vi "fgt get pressure channels Info.vi"(8 "error in (no error)":errorcluster) -> (0 "error out":errorcluster, 3 "Pressure channels info":T1[](array[typedef]) {"indexID" format="%.0x"; "index" format="%.0x"; "position" format="%.0x"; "DeviceSN" format="%.0x"; "firmware" format="%.0x"; "ControllerSN" format="%.0x"})   [LabVIEW 2020, in "fgt_SDK.lvlib"]
doc: "Get total number of initialized pressure channels. It is the sum of all MFCS, MFCS-EZ and FlowEZ pressure controllers"
uses:
  fgt_SDK.lvlib
  TypeDefs/fgt_CHANNEL_INFO.ctl
  TypeDefs/fgt_INSTRUMENT_TYPE.ctl
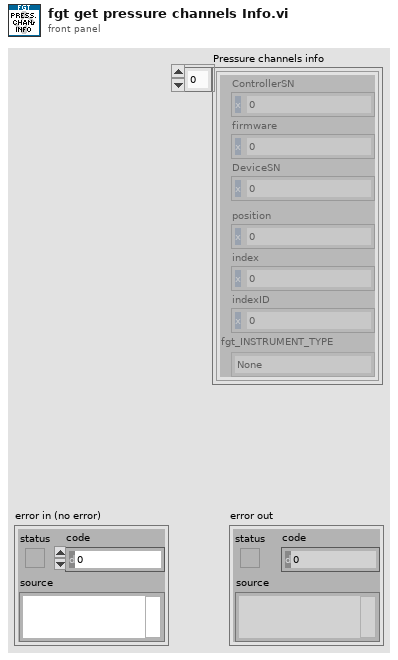
[diagram p1: front panel]
types:
  T1 = typedef "fgt_SDK.lvlib/fgt_CHANNEL_INFO.ctl" = cluster{"ControllerSN":u16, "firmware":u16, "DeviceSN":u16, "position":u32, "index":u32, "indexID":u32, "fgt_INSTRUMENT_TYPE":T2}
  T2 = typedef "fgt_SDK.lvlib/fgt_INSTRUMENT_TYPE.ctl" = enum32{"None", "MFCS", "MFCS_EZ", "FRP", "LineUP", "IPS"}
  T3 = cluster{"ControllerSN":u16, "firmware":u16, "DeviceSN":u16, "Padding":u16, "position":u32, "index":u32, "indexID":u32, "fgt_INSTRUMENT_TYPE":T2}
  T4 = cluster{"ControllerSN":u16, "firmware":u16, "DeviceSN":u16, "Padding":u16, "position":u32, "index":u32, "indexID":u32, "fgt_INSTRUMENT_TYPE":T2}[]
  T5 = typedef "fgt_SDK.lvlib/fgt_STATUS_INFO.ctl" = cluster{"InstrType":T2, "instrSN":u16, "errorCode":u8, "infoCode":u8, "detail":string}
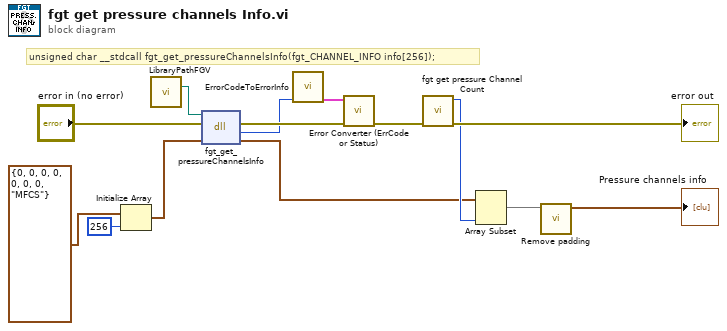
[diagram p0: block diagram]
diagram:
  # "unsigned char __stdcall fgt_get_pressureChannelsInfo(fgt_CHANNEL_INFO info[256]);"
  n1 = Initialize Array(T3 {"ControllerSN"=0, "firmware"=0, "DeviceSN"=0, "Padding"=0, "position"=0, "index"=0, "indexID"=0, "fgt_INSTRUMENT_TYPE"=enum."MFCS"} ("fgt_CHANNEL_INFO"), 256 ("dimension size")) -> (w8:T4)
  n2 = call "LibraryPathFGV.vi"() -> ("Path Out"=w1:path)  [unwired: 14 in, 1 out]
  n3 = dll-call lib="C:/Workspace/fgt-SDK/LabVIEW/dlls/fgt_SDK_*.*" fn="fgt_get_pressureChannelsInfo"(path in=w1, error in="error in (no error)", "info"=w8) -> (error out=w13:errorcluster, "return type"=w12:u8, "info"=w4:T4)  [unwired: 1 in, 1 out]
  n4 = call "ErrorCodeToErrorInfo.vi"("return type"=w12) -> ("StatusInfo"=w11:T5)  [unwired: 10 in]
  n5 = call "Error Converter (ErrCode or Status).vi"("error in (no error)"=w13, "StatusInfo"=w11) -> ("error out"=w7:errorcluster)  [unwired: 9 in]
  n6 = call "fgt get pressure Channel Count.vi"("error in (no error)"=w7) -> ("error out"=→"error out":errorcluster, "nbPChan out"=w5:u32)  [unwired: 9 in]
  n7 = Array Subset(array=w4, length=w5) -> (w2:T4)  [unwired: 1 in]
  n8 = call "Remove padding.vi"("Array in"=w2) -> ("Array out"=→"Pressure channels info":T1[])  [unwired: 10 in]
